vi "getNewValueXML.vi"(8 "error in (no error)":errorcluster, 11 "RampEvent in":refnum<class "RampEvent.lvclass">) -> (0 "error out":errorcluster, 2 "newValueXML":refnum<class "xmlNode.lvclass">, 3 "RampEvent out":refnum<class "RampEvent.lvclass">)   [LabVIEW 2011, in "Tools.lvlib" / "Scripting.lvlib" / "RampEvent.lvclass"]
uses:
  RampEvent.lvclass
  xmlNode/xmlNode.lvclass
  ScriptEvent.lvclass
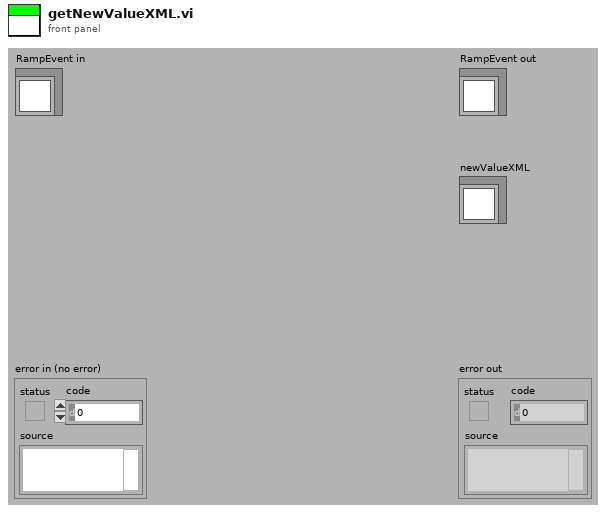
[diagram p1: front panel]
types:
  T1 = enum16{"time", "time_difference", "value", "frequency", "phase", "ramp_time", "value_step", "time_step", "number_of_steps", "start_value", "end_value", "start_freq", "start_amp", "start_phase", "end_freq", "end_amp", "end_phase"}
  T2 = cluster{"parameter_name":string, "parameter_value":string, "type":enum16{"time", "time_difference", "value", "frequency", "phase", "ramp_time", "value_step", "time_step", "number_of_steps", "start_value", "end_value", "start_freq", "start_amp", "start_phase", "end_freq", "end_amp", "end_phase"}}[]
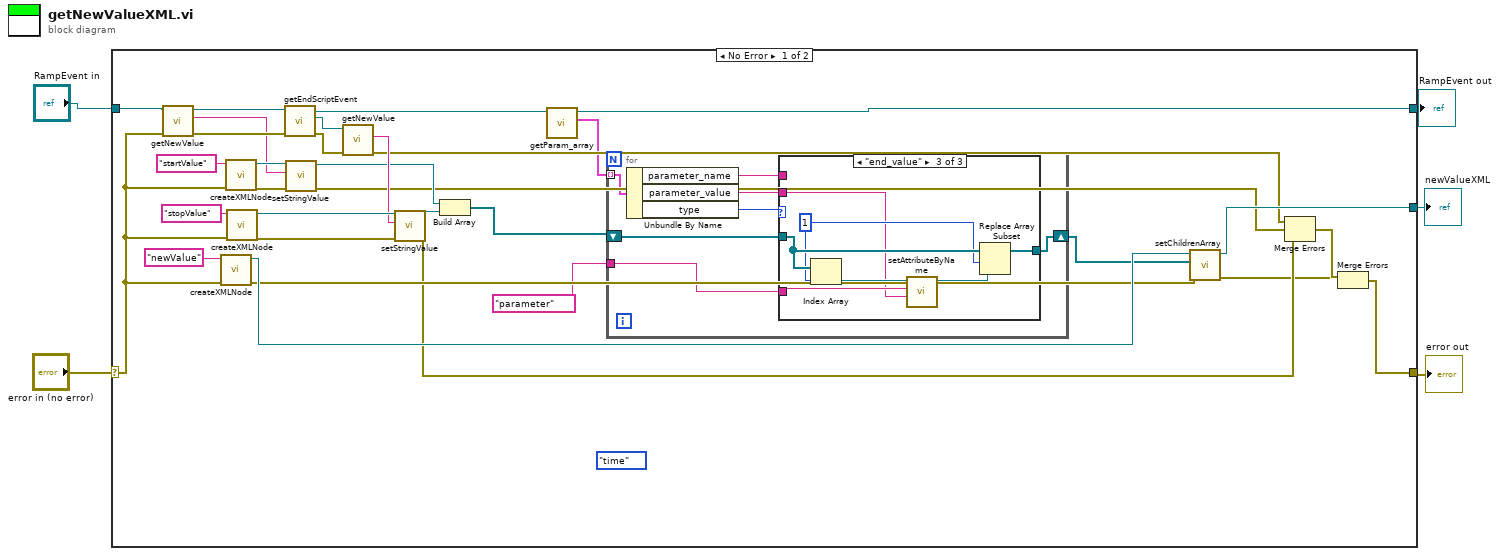
[diagram p0: block diagram]
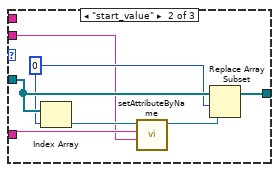
[diagram p3: hidden frame]
diagram:
  n1 = case shown="No Error" "error in (no error)" {
    selector: "error in (no error)" -> [w31 w61]
    tunnel: [w12 w61] -> w3
    tunnel: [w6 w60] -> w4
    tunnel: "RampEvent in" -> [w36 w60]
    tunnel: [w20 _] -> w1
    frame No Error {
      (unwired) T1."time" ("type")
      n2 = call "getNewValue.vi"("error in (no error)"=w31, "ScriptEvent.lvclass in"=w36) -> ("error out"=w34:errorcluster, "newValue"=w28:string, "ScriptEvent.lvclass out"=w35:refnum<class "RampEvent.lvclass">)  [unwired: 7 in]
      n3 = call "createXMLNode.vi"("error in (no error)"=w31, "name"="newValue") -> ("error out"=w21:errorcluster, "xmlNode out"=w22:refnum<class "xmlNode.lvclass">)  [unwired: 8 in]
      n4 = call "createXMLNode.vi"("error in (no error)"=w31, "name"="startValue") -> ("error out"=w29:errorcluster, "xmlNode out"=w30:refnum<class "xmlNode.lvclass">)  [unwired: 8 in]
      n5 = call "createXMLNode.vi"("error in (no error)"=w31, "name"="stopValue") -> ("error out"=w26:errorcluster, "xmlNode out"=w27:refnum<class "xmlNode.lvclass">)  [unwired: 8 in]
      n6 = call "getEndScriptEvent.vi"("error in (no error)"=w34, "RampEvent.lvclass in"=w35) -> ("error out"=w25:errorcluster, "ScriptEvent.lvclass"=w24:refnum<class "ScriptEvent.lvclass">, "RampEvent.lvclass out"=w7:refnum<class "RampEvent.lvclass">)  [unwired: 7 in]
      n7 = call-dynamic "setStringValue.vi"("error in (no error)"=w29, "stringValue"=w28, "xmlNode.lvclass in"=w30) -> ("error out"=w16:errorcluster, "xmlNode.lvclass out"=w19:refnum<class "xmlNode.lvclass">)  [unwired: 7 in]
      n8 = call "getNewValue.vi"("error in (no error)"=w25, "ScriptEvent.lvclass in"=w24) -> ("error out"=w17:errorcluster, "newValue"=w23:string)  [unwired: 7 in, 1 out]
      n9 = call-dynamic "setStringValue.vi"("error in (no error)"=w26, "stringValue"=w23, "xmlNode.lvclass in"=w27) -> ("error out"=w15:errorcluster, "xmlNode.lvclass out"=w18:refnum<class "xmlNode.lvclass">)  [unwired: 7 in]
      n10 = Build Array(w19, w18) -> (w9:refnum<class "xmlNode.lvclass">[])
      n11 = call "getParam_array.vi"("ScriptEvent in"=w7) -> ("param_array"=w10:T2, "ScriptEvent out"=w6:refnum<class "RampEvent.lvclass">)  [unwired: 8 in, 1 out]
      n12 = for {
        tunnel: w10 -> [w44] mode=indexing
        shift-right: [w39] -> w8
        shift-left: w9 -> [w42]
        tunnel: "parameter" -> [w38]
        n13 = Unbundle By Name(w44) -> ("parameter_name"=w41:string, "parameter_value"=w40:string, "type"=w43:T1)
        n14 = case shown="\"end_value\"" w43 {
          tunnel: w42 -> [w45 w50 w57]
          tunnel: w41 -> [_ _ _]
          tunnel: w40 -> [_ w46 w53]
          tunnel: [w45 w48 w55] -> w39
          tunnel: w38 -> [_ w47 w54]
          frame Default {
          }
          frame "start_value" {
            w49 = 0
            n15 = Index Array(array=w50, index=w49) -> (element=w52:refnum<class "xmlNode.lvclass">)
            n16 = call-dynamic "setAttributeByName.vi"("attributeValue"=w46, "attributeName"=w47, "xmlNode in"=w52) -> ("xmlNode out"=w51:refnum<class "xmlNode.lvclass">)  [unwired: 7 in, 1 out]
            n17 = Replace Array Subset(array=w50, new element=w51, index=w49) -> (w48:refnum<class "xmlNode.lvclass">[])
          }
          frame "end_value" {
            w56 = 1
            n18 = Index Array(array=w57, index=w56) -> (element=w59:refnum<class "xmlNode.lvclass">)
            n19 = call-dynamic "setAttributeByName.vi"("attributeValue"=w53, "attributeName"=w54, "xmlNode in"=w59) -> ("xmlNode out"=w58:refnum<class "xmlNode.lvclass">)  [unwired: 7 in, 1 out]
            n20 = Replace Array Subset(array=w57, new element=w58, index=w56) -> (w55:refnum<class "xmlNode.lvclass">[])
          }
        }
      }
      n21 = call-dynamic "setChildrenArray.vi"("error in (no error)"=w21, "Children"=w8, "xmlNode.lvclass in"=w22) -> ("error out"=w13:errorcluster, "xmlNode.lvclass out"=w20:refnum<class "xmlNode.lvclass">)  [unwired: 7 in]
      n22 = Merge Errors(w17, w16, w15) -> (w14:errorcluster)
      n23 = Merge Errors(w14, w13) -> (w12:errorcluster)
    }
    frame Error {
    }
  }
  "error out" <- w3
  "RampEvent out" <- w4
  "newValueXML" <- w1
